vi "waitForService.vi"(8 "error in (no error)":errorcluster, 11 "M1M3SAL in":refnum<class "M1M3SAL.lvclass">) -> (0 "error out":errorcluster, 3 "M1M3SAL out":refnum<class "M1M3SAL.lvclass">)   [LabVIEW 2016, in "M1M3SAL.lvlib" / "M1M3SAL.lvclass"]
uses:
  M1M3SAL.lvclass
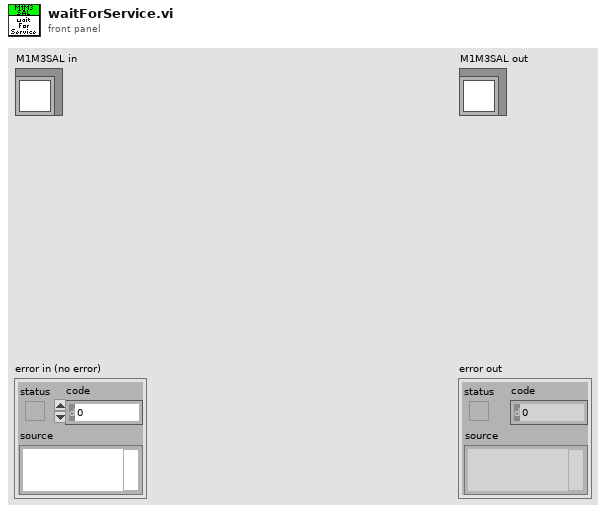
[diagram p1: front panel]
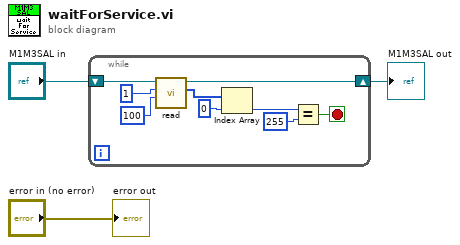
[diagram p0: block diagram]
diagram:
  n1 = while {
    shift-right: [w11] -> w2
    shift-left: "M1M3SAL in" -> [w12]
    stop <- w4 stop-if-true
    n2 = call "read.vi"("Timeout"=100, "NumberOfBytes"=1, "M1M3SAL in"=w12) -> ("Data"=w8:u8[], "M1M3SAL out"=w11:refnum<class "M1M3SAL.lvclass">)  [unwired: 6 in, 1 out]
    n3 = Index Array(array=w8, index=0) -> (element=w6:u8)
    n4 = Equal?(x=w6, y=u8 255) -> (x = y?=w4:bool)
  }
  "M1M3SAL out" <- w2
  "error out" <- "error in (no error)"
